vi "V-Meter Measure (2000).vi"(8 "error in (no error)":errorcluster, 11 "VISA resource name in":refnum<visa-resource-name>) -> (0 "error out":errorcluster, 2 "Measurement":dbl, 3 "VISA resource name out":refnum<visa-resource-name>)   [LabVIEW 2016, in "Hall Effect Library.lvlib"]
uses:
  Hall Effect Library.lvlib
  Global Variables/Test Settings.vi
  <instrlib>/Keithley 2000/Keithley 2000.lvlib
panel:
  out "Array":dbl[](array[numeric])
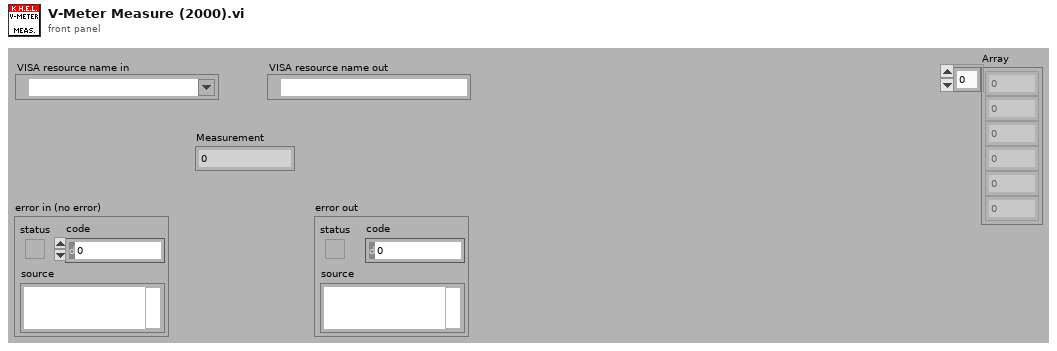
[diagram p1: front panel]
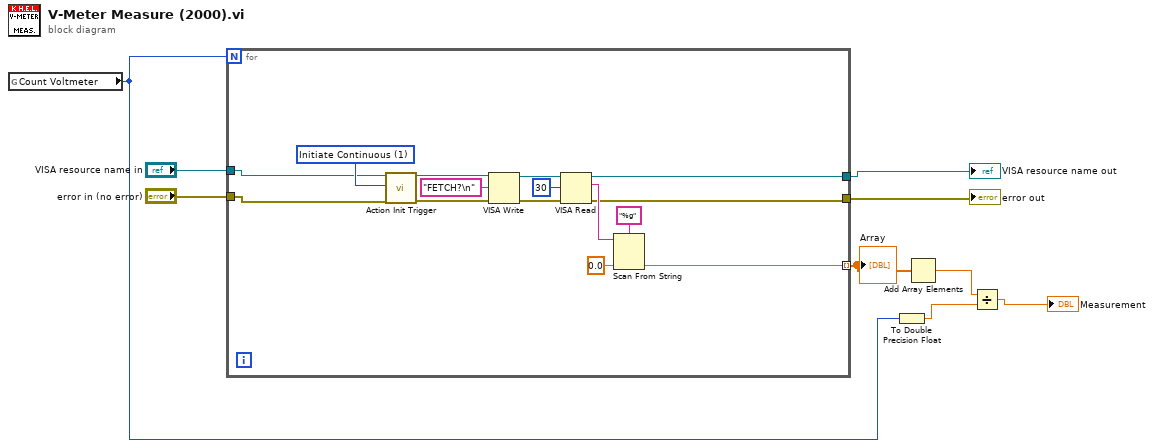
[diagram p0: block diagram]
diagram:
  n1 = global read "Test Settings.vi" "Count Voltmeter"() -> (w6:i32)
  n2 = for {
    N: w6 -> [_]
    tunnel: "VISA resource name in" -> [w14]
    tunnel: "error in (no error)" -> [w13]
    tunnel: [w12] -> w3
    tunnel: [w11] -> w2
    tunnel: [w10] -> w7 mode=indexing
    w15 = i16 1 items=["Don't Initiate"=-1, "Initiate Single"=0, "Initiate Continuous"=1] ("Inititiate Mode (1: Init Continuous)")
    n3 = call <instrlib>:"Action Init Trigger.vi"("VISA resource name"=w14, "Inititiate Mode (1: Init Continuous)"=w15, "error in (no error)"=w13) -> ("VISA resource name out"=w17:refnum<visa-resource-name>, "error out"=w16:errorcluster)  [unwired: 15 out]
    n4 = VISA Write(VISA resource name=w17, write buffer="FETCH?\n", error in (no error)=w16) -> (VISA resource name out=w19:refnum<visa-resource-name>, error out=w20:errorcluster)  [unwired: 1 out]
    n5 = VISA Read(VISA resource name=w19, byte count=u32 30, error in (no error)=w20) -> (VISA resource name out=w12:refnum<visa-resource-name>, read buffer=w22:string, error out=w11:errorcluster)  [unwired: 1 out]
    n6 = Scan From String(format string="%g", input string=w22, default 1=0.0 ("default value 1")) -> (output 1=w10:dbl)  [unwired: 2 in, 3 out]
  }
  "error out" <- w2
  "VISA resource name out" <- w3
  "Array" <- w7
  n7 = To Double Precision Float(number=w6) -> (double precision float=w4:dbl)
  n8 = Add Array Elements(numeric array=w7) -> (sum=w5:dbl)
  n9 = Divide(x=w5, y=w4) -> (x/y=→"Measurement":dbl)
